vi "Generate Modules Changed Event.vi"(8 "error in (no error)":errorcluster, 11 "Controller in":refnum<class "Controller.lvclass">) -> (0 "error out":errorcluster, 3 "Controller out":refnum<class "Controller.lvclass">)   [LabVIEW 2020, in "Controller.lvclass"]
uses:
  Controller.lvclass
  Controller.lvclass/Controller.ctl
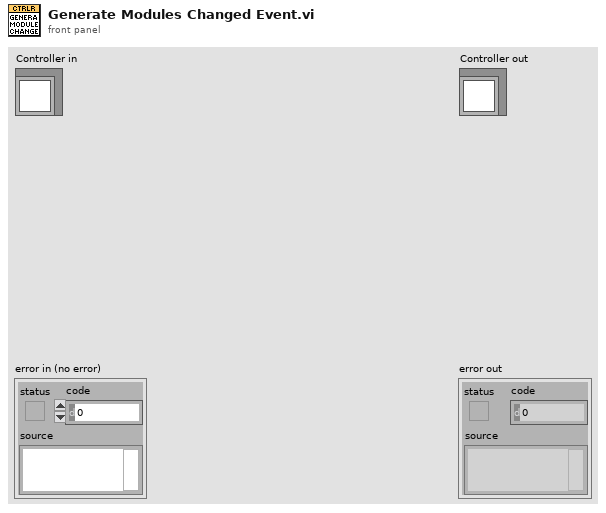
[diagram p1: front panel]
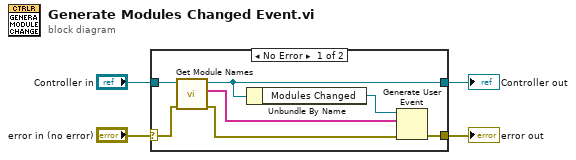
[diagram p0: block diagram]
diagram:
  n1 = case shown="No Error" "error in (no error)" {
    selector: "error in (no error)" -> [w6 w13]
    tunnel: [w10 w13] -> w3
    tunnel: [w8 w12] -> w1
    tunnel: "Controller in" -> [w9 w12]
    frame No Error {
      n2 = call "Get Module Names.vi"("error in (no error)"=w6, "Controller in"=w9) -> ("error out"=w5:errorcluster, "Names"=w7:string[], "Controller out"=w8:refnum<class "Controller.lvclass">)  [unwired: 7 in]
      n3 = Unbundle By Name(w8) -> ("Modules Changed"=w11:refnum<user-event>)
      n4 = Generate User Event(user event=w11, event data cluster=w7, error in=w5) -> (error out=w10:errorcluster)  [unwired: 1 in, 1 out]
    }
    frame Error {
    }
  }
  "error out" <- w3
  "Controller out" <- w1
